vi "pattern_match+matching_decay+direction&boudning_box.vi"(0 "Imaginea":path, 1 "Template":path) -> (13 "y 2":sgl, 14 "Directia":i32, 15 "x":sgl, 17 "y":sgl, 18 "x 2":sgl, 19 "Image":T1(plugin-control))   [LabVIEW 2015]
uses:
  <vilib>/imath/engines/lvmath2/RunTimeEngine/NodeEndStatement/NIMS_NodeEndStatement_Output.vi
  <instcachedir>/0/NIMS_NodeEndStatement_Output_53EC0D466D134D7ABD903AC30B43404B.lvgen/NIMS_NodeEndStatement_Output_53EC0D466D134D7ABD903AC30B43404B_010.vi
  <vilib>/imath/engines/lvmath2/RunTimeEngine/ErrorHandling/NIMS_Finalize Error.vi
panel:
  out "Image 2":T1(plugin-control)
  out "Angle":sgl
  out "element":T2
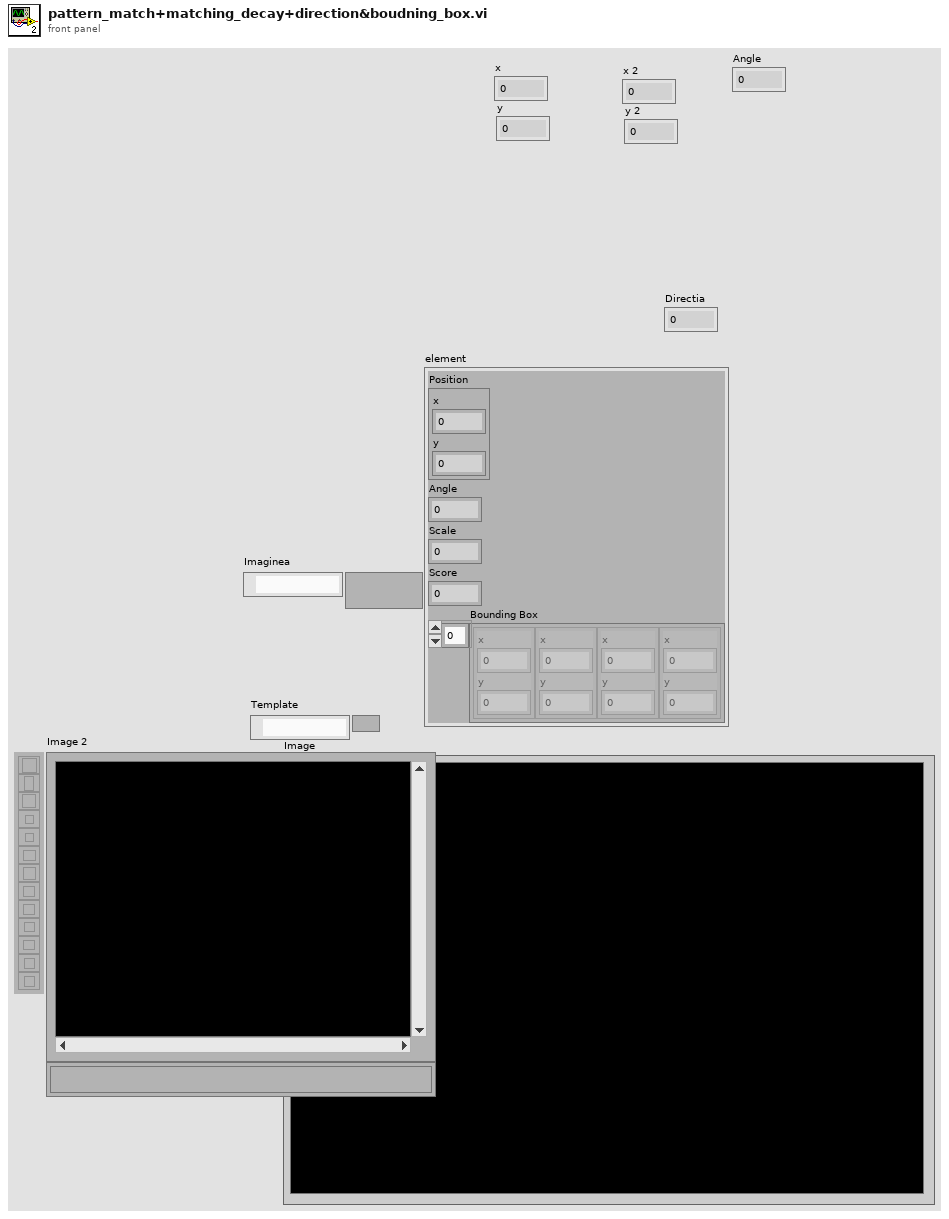
[diagram p1: front panel]
types:
  T1 = typedef "IMAQ Image.ctl" = refnum<image>
  T2 = cluster{"Position":cluster{"x":sgl, "y":sgl}, "Angle":sgl, "Scale":sgl, "Score":sgl, "Bounding Box":cluster{"x":sgl, "y":sgl}[]}
  T3 = cluster{"Position":cluster{"x":sgl, "y":sgl}, "Angle":sgl, "Scale":sgl, "Score":sgl, "Bounding Box":cluster{"x":sgl, "y":sgl}[]}[]
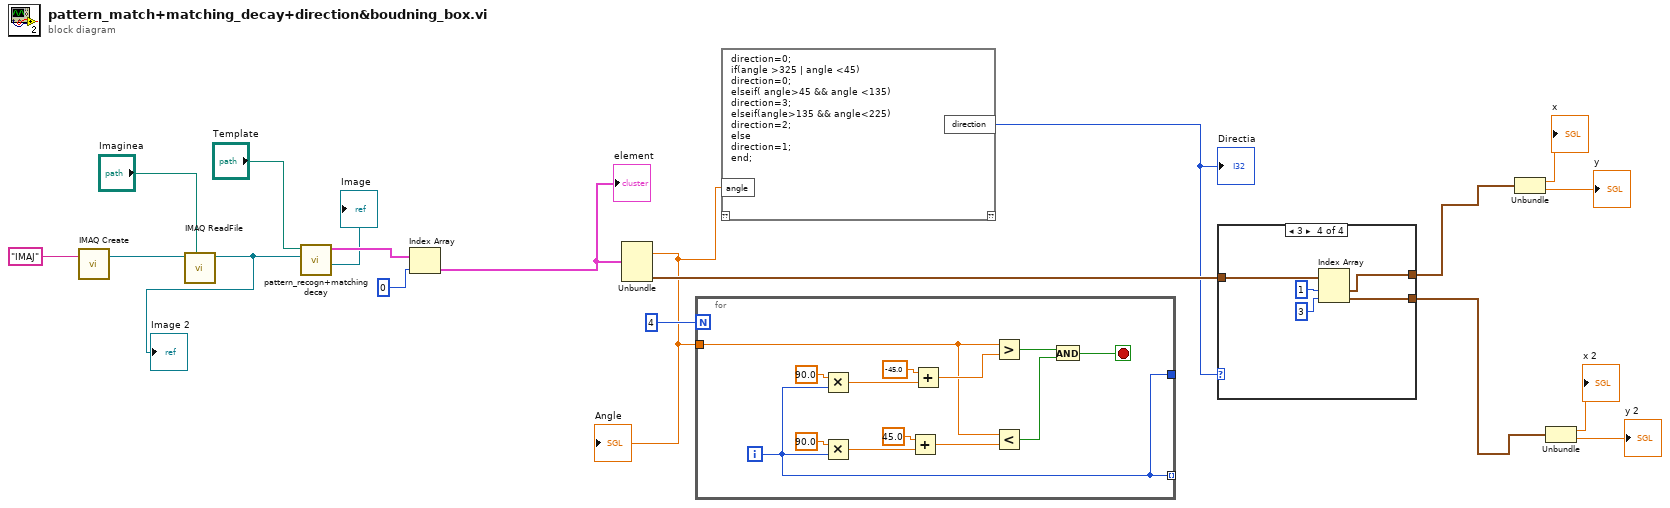
[diagram p0: block diagram]
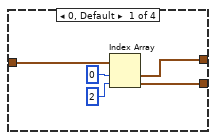
[diagram p2: hidden frame]
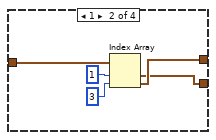
[diagram p3: hidden frame]
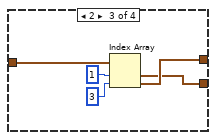
[diagram p4: hidden frame]
diagram:
  n1 = call "IMAQ Create"("Image Name"="IMAJ") -> ("New Image"=w19:T1)  [unwired: 4 in, 1 out]
  n2 = call "IMAQ ReadFile"("File Path"="Imaginea", "Image"=w19) -> ("Image Out"=w3:T1)  [unwired: 5 in, 4 out]
  "Image 2" <- w3
  n3 = call "pattern_recogn+matching decay.vi"("Image Out"=w3, "Path 3"="Template") -> ("Image"=→"Image":T1, "Matches (pixel)"=w15:T3)  [unwired: 7 in, 1 out]
  n4 = Index Array(array=w15, index=0) -> (element=w12:T2)
  "element" <- w12
  n5 = Unbundle(w12) -> ("Angle"=w2:sgl, "Bounding Box"=w10:cluster{"x":sgl, "y":sgl}[])  [unwired: 3 out]
  "Angle" <- w2
  n6 = for {
    N: 4 -> [_]
    tunnel: w2 -> [w26]
    tunnel: [w21] -> _
    tunnel: [w21] -> _ mode=indexing
    i -> [w21]
    stop <- w23 stop-if-true
    n7 = Multiply(x=sgl 90.0, y=w21) -> (x*y=w30:sgl)
    n8 = Multiply(x=sgl 90.0, y=w21) -> (x*y=w20:sgl)
    n9 = Add(x=sgl 45.0, y=w20) -> (x+y=w27:sgl)
    n10 = Add(x=sgl -45.0, y=w30) -> (x+y=w29:sgl)
    n11 = Greater?(x=w26, y=w29) -> (0:w25:bool)
    n12 = Less?(x=w26, y=w27) -> (x < y?=w24:bool)
    n13 = And(x=w25, y=w24) -> (x .and. y?=w23:bool)
  }
  n14 = mathscript code="direction=0;\nif(angle >325 | angle <45)\ndirection=0;\nelseif( angle>45 && angle <135)\ndirection=3;\nelseif(angle>135 && angle<225)\ndirection=2;\nelse\ndirection=1;\nend;"("angle"=w2) -> ("direction"=w1:i32)  [unwired: 1 in, 1 out]
  "Directia" <- w1
  n15 = case shown="3" w1 {
    tunnel: w10 -> [w37 w40 w45 w50]
    tunnel: [w34 w39 w44 w49] -> w9
    tunnel: [w33 w38 w43 w48] -> w4
    frame 0, Default {
      n16 = Index Array(array=w37, index #1=0 ("index"), index #2=2 ("index")) -> (element #1=w34:cluster{"x":sgl, "y":sgl}, element #2=w33:cluster{"x":sgl, "y":sgl})
    }
    frame 1 {
      n17 = Index Array(array=w40, index #1=1 ("index"), index #2=3 ("index")) -> (element #1=w38:cluster{"x":sgl, "y":sgl}, element #2=w39:cluster{"x":sgl, "y":sgl})
    }
    frame 2 {
      n18 = Index Array(array=w45, index #1=1 ("index"), index #2=3 ("index")) -> (element #1=w43:cluster{"x":sgl, "y":sgl}, element #2=w44:cluster{"x":sgl, "y":sgl})
    }
    frame 3 {
      n19 = Index Array(array=w50, index #1=1 ("index"), index #2=3 ("index")) -> (element #1=w49:cluster{"x":sgl, "y":sgl}, element #2=w48:cluster{"x":sgl, "y":sgl})
    }
  }
  n20 = Unbundle(w9) -> ("x"=→"x":sgl, "y"=→"y":sgl)
  n21 = Unbundle(w4) -> ("x"=→"x 2":sgl, "y"=→"y 2":sgl)
